vi "NewDataInBuffer_Parse.vi"(8 "error in (no error)":errorcluster, 11 "Message":variant) -> (0 "error out":errorcluster, 2 "buffer location":u32, 3 "data group":string)   [LabVIEW 2017, in "DataAccumulator.lvlib"]
uses:
  <vilib>/addons/InsightCM/Devices/Shared/Common/DataAccumulator/DataAccumulator.lvlib
  <vilib>/addons/InsightCM/Devices/Shared/Common/DataAccumulator/controls/NewDataInBuffer.ctl
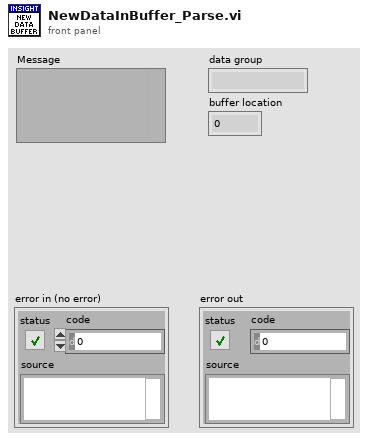
[diagram p1: front panel]
types:
  T1 = typedef "DataAccumulator.lvlib/NewDataInBuffer.ctl" = cluster{"DataGroup":string, "buffer location":u32}
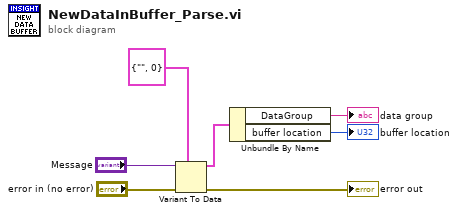
[diagram p0: block diagram]
diagram:
  n1 = Variant To Data(error in="error in (no error)", type=T1 {"DataGroup"="", "buffer location"=0}, Variant="Message") -> (data=w4:T1, error out=→"error out":errorcluster)
  n2 = Unbundle By Name(w4) -> ("DataGroup"=→"data group":string, "buffer location"=→"buffer location":u32)
